vi "Simple UDP - Sender.vi"() -> ()   [LabVIEW 2016]
doc: "The UDP protocol differs from TCP in that there is no error-checking with the packets of information that are sent, and thus no guarantee whatsoever that an intended recipient will actually receive a given piece of data.\n\nUDP does offer the ability to \"broadcast\" data across a network--simply specify an IP Address of all ones (255.255.255.255) to attempt to broadcast information network-wide. Keep in mind that routers and other network hardware will generally refuse to forward the broadcast beyond certain points, so the extent of the broadcast will in practice be limited."
uses:
  <vilib>/userdefined/High Color/IMAQdx.ctl
  <vilib>/vision/driver/NI_Vision_Acquisition_Software.lvlib
panel:
  out "FileString":string
  out "Image":T1(plugin-control)
  in  "Camera Name":T2="cam0"
  in  "Stop":bool
  # "Overview: Demonstrates the use of the UDP functions to send data over a UDP connection.\nInstructions:\n1. Run the VI.\n2. Open Simple UDP - Receiver.vi and follow the instructions on its front panel.\n3. Click Stop to stop the VI."
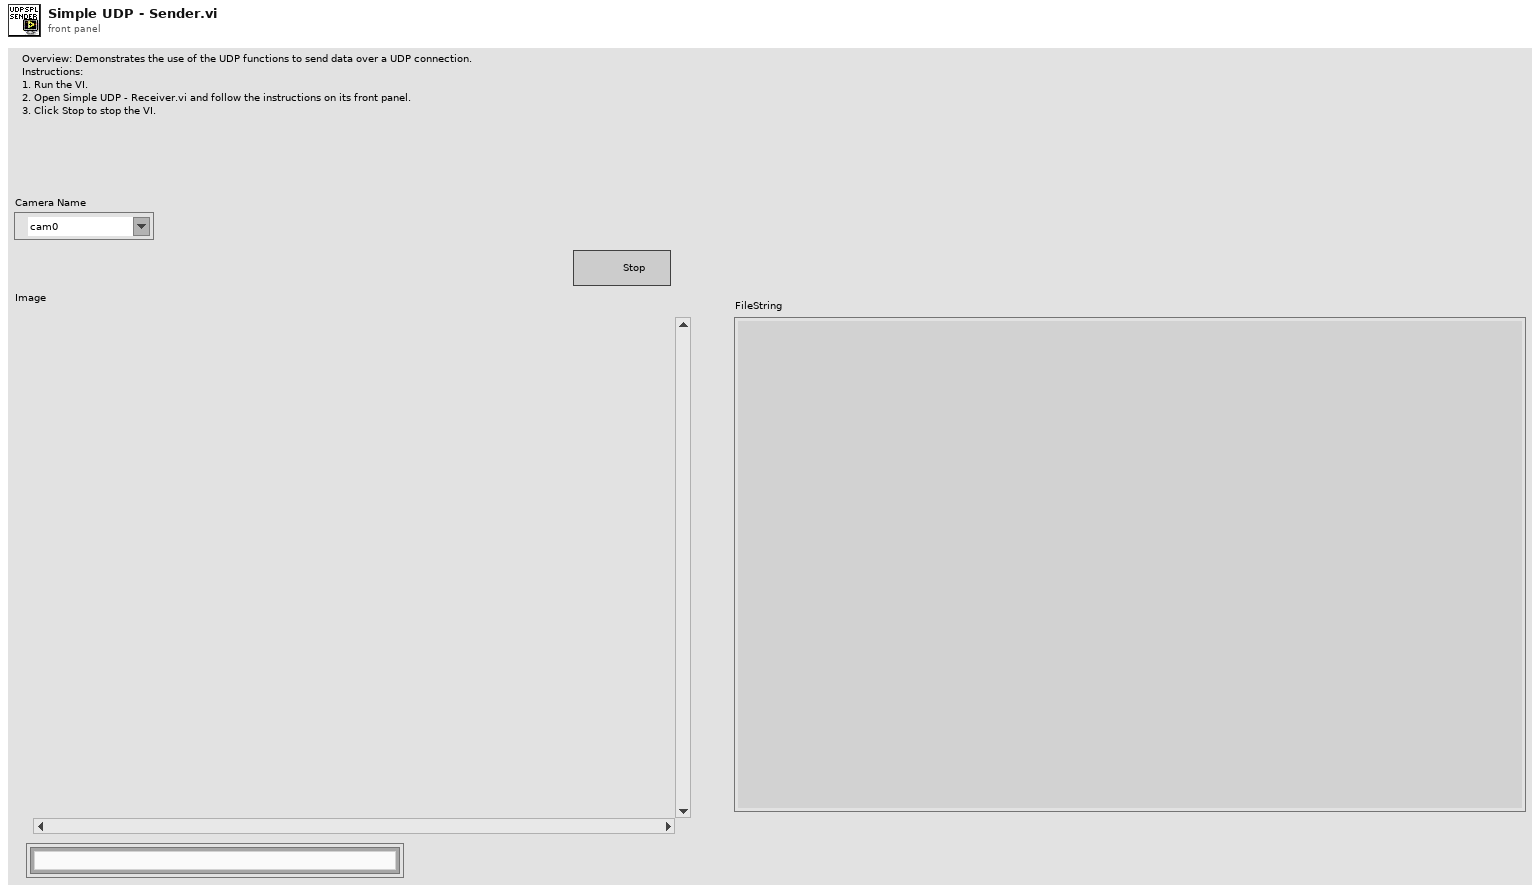
[diagram p1: front panel]
types:
  T1 = typedef "IMAQ Image.ctl" = refnum<image>
  T2 = typedef "IMAQdx.ctl" = refnum<k21>
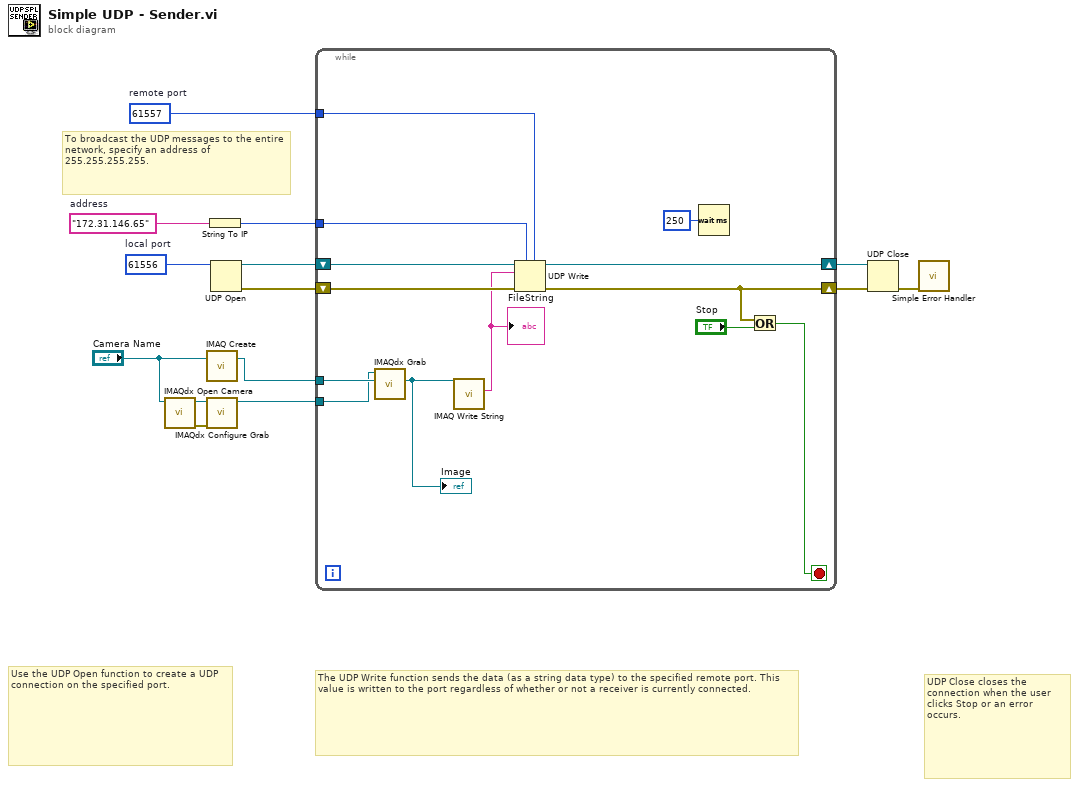
[diagram p0: block diagram]
diagram:
  w6 = u16 61557  # remote port
  w7 = u16 61556  # local port
  w12 = "172.31.146.65"  # address
  # "To broadcast the UDP messages to the entire network, specify an address of 255.255.255.255."
  # "UDP Close closes the connection when the user clicks Stop or an error occurs."
  # "The UDP Write function sends the data (as a string data type) to the specified remote port. This value is written to the port regardless of whether or not a receiver is currently connected."
  # "Use the UDP Open function to create a UDP connection on the specified port."
  n1 = call <vilib>:"IMAQdx Open Camera.vi"("Session In"="Camera Name") -> ("error out"=w3:errorcluster, "Session Out"=w4:T2)  [unwired: 2 in, 7 out]
  n2 = call "IMAQ Create"("Image Name"="Camera Name") -> ("New Image"=w2:T1)  [unwired: 3 in, 2 out]
  n3 = call <vilib>:"IMAQdx Configure Grab.vi"("error in"=w3, "Session In"=w4) -> ("Session Out"=w1:T2)  [unwired: 9 out]
  n4 = String To IP(1:w12) -> (0:w10:u32)
  n5 = UDP Open(11:w7) -> (port=w9:refnum<k16>, 0:w8:errorcluster)  [unwired: 4 in, 1 out]
  n6 = while {
    tunnel: w10 -> [w25]
    tunnel: w6 -> [w22]
    tunnel: w2 -> [w21]
    tunnel: w1 -> [w20]
    shift-right: [w27] -> w14
    shift-left: w9 -> [w24]
    shift-right: [w26] -> w13
    shift-left: w8 -> [w23]
    stop <- w15 stop-if-true
    n7 = call <vilib>:"IMAQdx Grab.vi"("Image In"=w21, "Session In"=w20) -> ("Image Out"=w17:T1)  [unwired: 2 in, 7 out]
    "Image" <- w17
    n8 = call-poly "IMAQ Write String"("Image"=w17) -> ("FileString"=w16:string)  [unwired: 8 in, 2 out]
    "FileString" <- w16
    n9 = UDP Write(address=w25, port or service name=w22, connection ID=w24, data in=w16, 8:w23) -> (error out=w26:errorcluster, 3:w27:refnum<k16>)  [unwired: 1 in]
    n10 = Wait (ms)(milliseconds to wait=u32 250) -> ()  [unwired: 1 out]
    n11 = Or(x=w26, y="Stop") -> (x .or. y?=w15:bool)
  }
  n12 = UDP Close(connection ID=w14, 8:w13) -> (error out=w11:errorcluster)  [unwired: 1 out]
  n13 = call <vilib>:"Simple Error Handler.vi"("error in (no error)"=w11) -> ()  [unwired: 4 in, 5 out]
